vi "Phased array GUI.vi"() -> ()   [LabVIEW 2020]
uses:
  <vilib>/Instr/_visa.llb/Select Event Type.ctl
  Devices/Controls/Register to Write.ctl
  <vilib>/Instr/_visa.llb/VISA Configure Serial Port (Instr).vi
  <vilib>/Utility/file.llb/Read Delimited Spreadsheet (string).vi
  Devices/PIC-device/PIC-Device.lvclass
panel:
  out "Array 2":string[][](array[string])
  out "Array":string[](array[string])
  in  "System Open Button":bool
  in  "Calibration data (hex)":string[][](array[string])=[["0", "1", "0", "1"], ["F", "0", "D", "0"], ["C", "6", "E", "4"], ["3", "0", "2", "0"], ["8", "3", "B", "0"], ["C", "6", "8", "8"], ["4", "0", "1", "0"], ["8", "3", "8", "3"], ["D", "7", "C", "8"], ["4", "0", "1", "1"], ["8", "3", "D", "0"], ["B", "7", "9", "A"]]
  in  "COM-port U5 & U7":refnum<visa-resource-name>
  in  "COM-port U1 & U3":refnum<visa-resource-name>
  in  "System Stop Button":bool
  in  "U3 setting":i32(slide) min=0 max=180 step=90 scale=0.0..180.0
  in  "U7 setting":i32(slide) min=0 max=180 step=90 scale=0.0..180.0
  in  "U5 setting":i32(slide) min=0 max=180 step=90 scale=0.0..180.0
  in  "U1 setting":i32(slide) min=0 max=180 step=90 scale=0.0..180.0
  in  "Setting":i32[][](array[numeric])=[[1, 0, 0, 0, 0, 0], [1, 90, 0, 0, 0, 0], [1, 180, 0, 0, 0, 0], [3, 0, 0, 0, 0, 0], [3, 90, 0, 0, 0, 0], [3, 180, 0, 0, 0, 0], [5, 0, 0, 0, 0, 0], [5, 90, 0, 0, 0, 0], [5, 180, 0, 0, 0, 0], [7, 0, 0, 0, 0, 0], [7, 90, 0, 0, 0, 0], [7, 180, 0, 0, 0, 0]]
  # "Ux     angle    C1     C2     C3     C4"
  # "U1"
  # "U5"
  # "U3"
  # "U7"
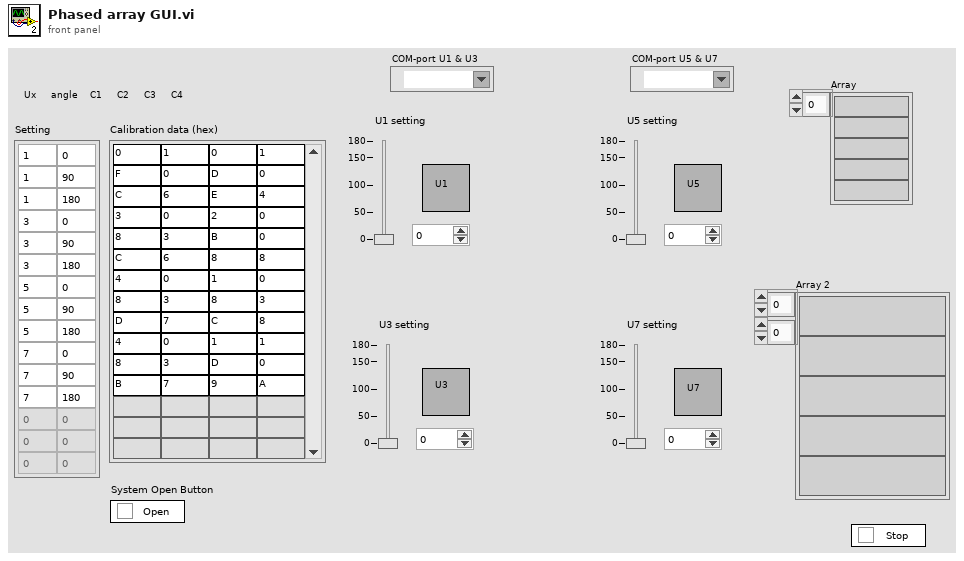
[diagram p1: front panel]
types:
  T1 = typedef "Select Event Type.ctl" = u32
  T2 = typedef "PIC-Device.lvclass/Register to Write.ctl" = cluster{"Register":u32, "Value":u32, "Dev Address":u32, "Physical Adress":u32}
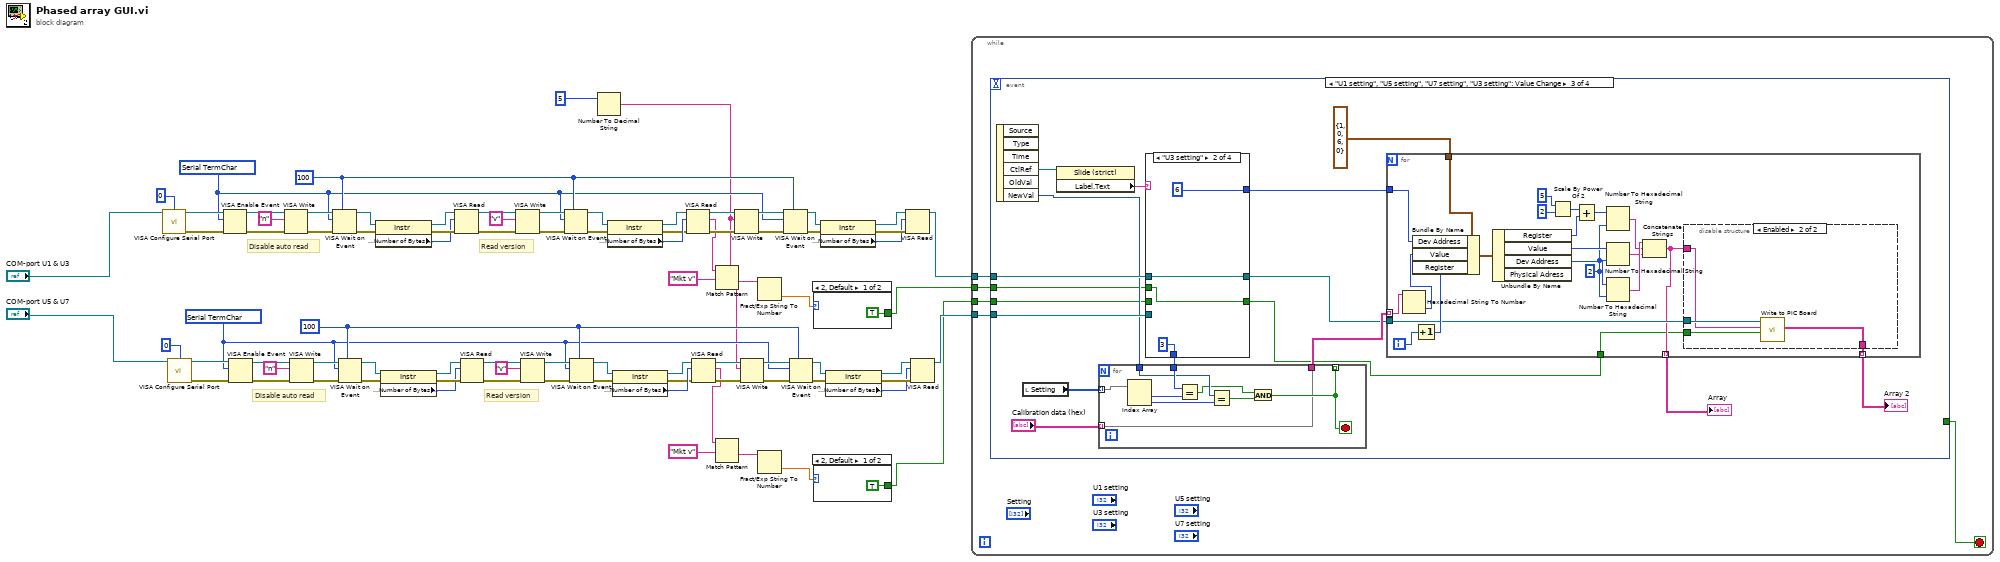
[diagram p0: block diagram]
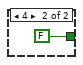
[diagram p2: hidden frame]
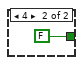
[diagram p3: hidden frame]
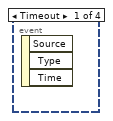
[diagram p4: hidden frame]
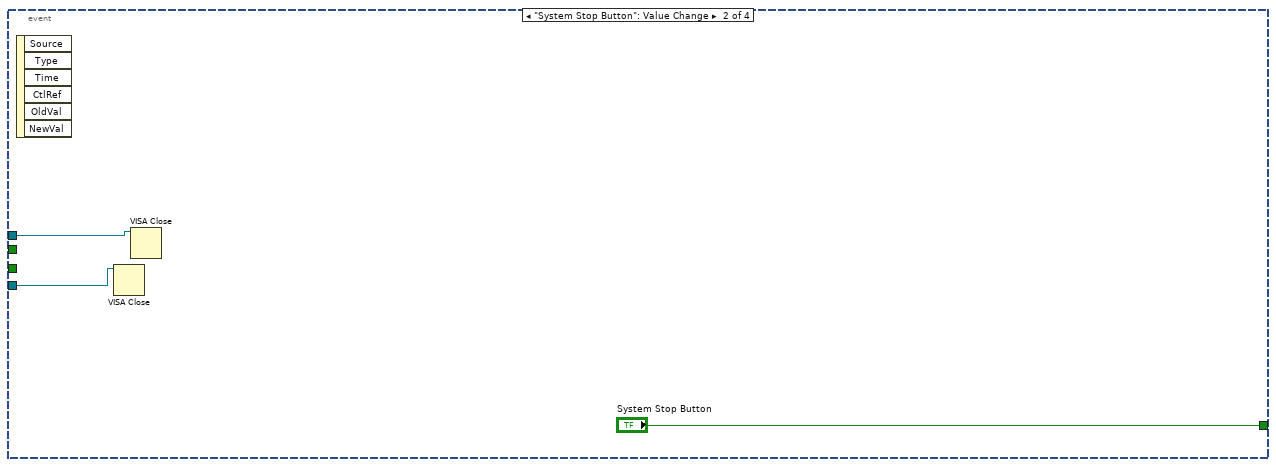
[diagram p5: hidden frame]
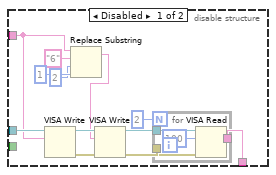
[diagram p6: hidden frame]
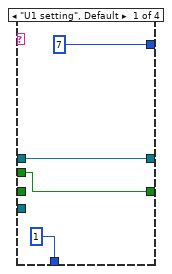
[diagram p7: hidden frame]
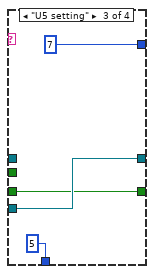
[diagram p8: hidden frame]
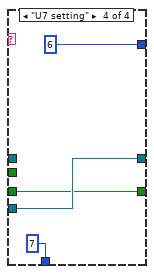
[diagram p9: hidden frame]
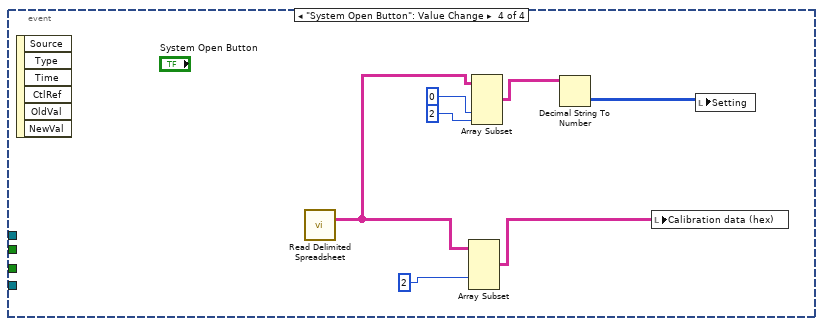
[diagram p10: hidden frame]
diagram:
  w18 = u32 100 ("timeout (0)")
  w17 = T1 1073684516 items=["Service Request"=1073684491, "Trigger"=3221168138, "Clear"=1073684493, "VXI Signal"=1073684512, "VXI/VME Interrupt"=3221168161, "VXI/VME Sysfail"=1073684509, "VXI/VME Sysreset"=1073684510, "GPIB CIC"=1073684498, "GPIB Talk"=1073684499, "GPIB Listen"=1073684500, "PXI Interrupt"=1073684514, "Serial Break"=1073684515, "Serial TermChar"=1073684516, "Serial CTS"=1073684521, "Serial DSR"=1073684522, "Serial DCD"=1073684524, "Serial RI"=1073684526, "Serial Character"=1073684533, "USB Interrupt"=1073684535, "All Enabled"=1073709055] ("Event Type")
  w52 = u32 100 ("timeout (0)")
  w51 = T1 1073684516 items=["Service Request"=1073684491, "Trigger"=3221168138, "Clear"=1073684493, "VXI Signal"=1073684512, "VXI/VME Interrupt"=3221168161, "VXI/VME Sysfail"=1073684509, "VXI/VME Sysreset"=1073684510, "GPIB CIC"=1073684498, "GPIB Talk"=1073684499, "GPIB Listen"=1073684500, "PXI Interrupt"=1073684514, "Serial Break"=1073684515, "Serial TermChar"=1073684516, "Serial CTS"=1073684521, "Serial DSR"=1073684522, "Serial DCD"=1073684524, "Serial RI"=1073684526, "Serial Character"=1073684533, "USB Interrupt"=1073684535, "All Enabled"=1073709055] ("Event Type")
  # "Read version"
  # "Disable auto read"
  # "Read version"
  # "Disable auto read"
  n1 = call-poly "VISA Configure Serial Port"("VISA resource name"="COM-port U1 & U3", "termination char\n(0xA = '\\n' = LF)"=u8 0 ("termination char\n(0xA = '\\n' = LF)")) -> ("VISA resource name out"=w48:refnum<visa-resource-name>, "error out"=w49:errorcluster)  [unwired: 12 in]
  n2 = call-poly "VISA Configure Serial Port"("VISA resource name"="COM-port U5 & U7", "termination char\n(0xA = '\\n' = LF)"=u8 0 ("termination char\n(0xA = '\\n' = LF)")) -> ("VISA resource name out"=w82:refnum<visa-resource-name>, "error out"=w83:errorcluster)  [unwired: 12 in]
  n3 = VISA Enable Event(8:w49, 10:w17, 11:w48) -> (0:w47:errorcluster, 3:w46:refnum<visa-resource-name>)  [unwired: 1 in]
  n4 = VISA Enable Event(8:w83, 10:w51, 11:w82) -> (0:w81:errorcluster, 3:w80:refnum<visa-resource-name>)  [unwired: 1 in]
  n5 = VISA Write(VISA resource name=w46, write buffer="n", error in (no error)=w47) -> (VISA resource name out=w43:refnum<visa-resource-name>, error out=w44:errorcluster)  [unwired: 1 out]
  n6 = VISA Write(VISA resource name=w80, write buffer="n", error in (no error)=w81) -> (VISA resource name out=w77:refnum<visa-resource-name>, error out=w78:errorcluster)  [unwired: 1 out]
  n7 = VISA Wait on Event(7:w18, 8:w44, 10:w17, 11:w43) -> (0:w41:errorcluster, 3:w42:refnum<visa-resource-name>)  [unwired: 1 in, 2 out]
  n8 = VISA Wait on Event(7:w52, 8:w78, 10:w51, 11:w77) -> (0:w75:errorcluster, 3:w76:refnum<visa-resource-name>)  [unwired: 1 in, 2 out]
  n9 = property class="Instr"(reference=w42, error in=w41) -> (reference out=w38:refnum<visa-resource-name>, error out=w40:errorcluster, "Serial Settings:Number of Bytes at Serial Port"=w39:u32)
  n10 = property class="Instr"(reference=w76, error in=w75) -> (reference out=w72:refnum<visa-resource-name>, error out=w74:errorcluster, "Serial Settings:Number of Bytes at Serial Port"=w73:u32)
  n11 = VISA Read(VISA resource name=w38, byte count=w39, error in (no error)=w40) -> (VISA resource name out=w22:refnum<visa-resource-name>, error out=w21:errorcluster)  [unwired: 2 out]
  n12 = VISA Read(VISA resource name=w72, byte count=w73, error in (no error)=w74) -> (VISA resource name out=w56:refnum<visa-resource-name>, error out=w55:errorcluster)  [unwired: 2 out]
  n13 = VISA Write(VISA resource name=w22, write buffer="v", error in (no error)=w21) -> (VISA resource name out=w25:refnum<visa-resource-name>, error out=w24:errorcluster)  [unwired: 1 out]
  n14 = VISA Write(VISA resource name=w56, write buffer="v", error in (no error)=w55) -> (VISA resource name out=w59:refnum<visa-resource-name>, error out=w58:errorcluster)  [unwired: 1 out]
  n15 = VISA Wait on Event(7:w18, 8:w24, 10:w17, 11:w25) -> (0:w27:errorcluster, 3:w26:refnum<visa-resource-name>)  [unwired: 1 in, 2 out]
  n16 = VISA Wait on Event(7:w52, 8:w58, 10:w51, 11:w59) -> (0:w61:errorcluster, 3:w60:refnum<visa-resource-name>)  [unwired: 1 in, 2 out]
  n17 = Number To Decimal String(number=5) -> (decimal integer string=w11:string)  [unwired: 1 in]
  n18 = property class="Instr"(reference=w26, error in=w27) -> (reference out=w30:refnum<visa-resource-name>, error out=w28:errorcluster, "Serial Settings:Number of Bytes at Serial Port"=w29:u32)
  n19 = property class="Instr"(reference=w60, error in=w61) -> (reference out=w64:refnum<visa-resource-name>, error out=w62:errorcluster, "Serial Settings:Number of Bytes at Serial Port"=w63:u32)
  n20 = VISA Read(VISA resource name=w30, byte count=w29, error in (no error)=w28) -> (VISA resource name out=w19:refnum<visa-resource-name>, read buffer=w3:string, error out=w20:errorcluster)  [unwired: 1 out]
  n21 = VISA Read(VISA resource name=w64, byte count=w63, error in (no error)=w62) -> (VISA resource name out=w53:refnum<visa-resource-name>, read buffer=w7:string, error out=w54:errorcluster)  [unwired: 1 out]
  n22 = Match Pattern(string=w3, regular expression="Mkt v" ("format string")) -> (after substring=w5:string)  [unwired: 1 in, 3 out]
  n23 = Match Pattern(string=w7, regular expression="Mkt v" ("format string")) -> (after substring=w9:string)  [unwired: 1 in, 3 out]
  n24 = VISA Write(VISA resource name=w19, write buffer=w11, error in (no error)=w20) -> (VISA resource name out=w36:refnum<visa-resource-name>, error out=w37:errorcluster)  [unwired: 1 out]
  n25 = VISA Write(VISA resource name=w53, write buffer=w11, error in (no error)=w54) -> (VISA resource name out=w70:refnum<visa-resource-name>, error out=w71:errorcluster)  [unwired: 1 out]
  n26 = Fract/Exp String To Number(string=w5) -> (number=w6:dbl)  [unwired: 3 in, 1 out]
  n27 = Fract/Exp String To Number(string=w9) -> (number=w8:dbl)  [unwired: 3 in, 1 out]
  n28 = VISA Wait on Event(7:w18, 8:w37, 10:w17, 11:w36) -> (0:w34:errorcluster, 3:w35:refnum<visa-resource-name>)  [unwired: 1 in, 2 out]
  n29 = VISA Wait on Event(7:w52, 8:w71, 10:w51, 11:w70) -> (0:w68:errorcluster, 3:w69:refnum<visa-resource-name>)  [unwired: 1 in, 2 out]
  n30 = case shown="2, Default" w6 {
    tunnel: [TRUE FALSE] -> w2
    frame 2, Default {
    }
    frame 4 {
    }
  }
  n31 = case shown="2, Default" w8 {
    tunnel: [TRUE FALSE] -> w1
    frame 2, Default {
    }
    frame 4 {
    }
  }
  n32 = property class="Instr"(reference=w35, error in=w34) -> (reference out=w31:refnum<visa-resource-name>, error out=w33:errorcluster, "Serial Settings:Number of Bytes at Serial Port"=w32:u32)
  n33 = property class="Instr"(reference=w69, error in=w68) -> (reference out=w65:refnum<visa-resource-name>, error out=w67:errorcluster, "Serial Settings:Number of Bytes at Serial Port"=w66:u32)
  n34 = VISA Read(VISA resource name=w31, byte count=w32, error in (no error)=w33) -> (VISA resource name out=w13:refnum<visa-resource-name>)  [unwired: 3 out]
  n35 = VISA Read(VISA resource name=w65, byte count=w66, error in (no error)=w67) -> (VISA resource name out=w14:refnum<visa-resource-name>)  [unwired: 3 out]
  n36 = while {
    tunnel: w13 -> [w92]
    tunnel: w14 -> [w91]
    tunnel: w2 -> [w90]
    tunnel: w1 -> [w89]
    stop <- w93 stop-if-true
    n37 = event shown="[2] \"U1 setting\", \"U5 setting\", \"U7 setting\", \"U3 setting\": Value Change" {
      selector: _ -> [_ _ _ _]
      dyn-events: _ -> [_ _ _ _]
      timeout: _ -> [_ _ _ _]
      tunnel: [_ "System Stop Button" _ _] -> w93
      tunnel: w92 -> [_ w95 w111 _]
      tunnel: w91 -> [_ w94 w110 _]
      tunnel: w90 -> [_ _ w99 _]
      tunnel: w89 -> [_ _ w98 _]
      event Timeout {
        n38 = event-data() -> ()  [unwired: 1 in, 3 out]
      }
      event "System Stop Button": Value Change {
        n39 = event-data() -> ()  [unwired: 1 in, 6 out]
        n40 = VISA Close(VISA resource name=w94) -> ()  [unwired: 1 in, 1 out]
        n41 = VISA Close(VISA resource name=w95) -> ()  [unwired: 1 in, 1 out]
      }
      event "U1 setting", "U5 setting", "U7 setting", "U3 setting": Value Change {
        n42 = event-data() -> ("CtlRef"=w113:refnum<vi>, "NewVal"=w107:i32)  [unwired: 1 in, 4 out]
        n43 = local read "Setting"() -> (w109:i32[][])
        n44 = property class="Slide (strict)"(reference=w113) -> ("Label.Text"=w112:string)  [unwired: 1 in, 2 out]
        n45 = case shown="\"U3 setting\"" w112 {
          tunnel: [w168 w172 w175 w179] -> w102
          tunnel: w111 -> [w168 w172 _ _]
          tunnel: [u32 7 ("Dev Address") u32 6 ("Dev Address") u32 7 ("Dev Address") u32 6 ("Dev Address")] -> w103
          tunnel: w110 -> [_ _ w175 w179]
          tunnel: [1 3 5 7] -> w108
          tunnel: w99 -> [w165 w169 _ _]
          tunnel: w98 -> [_ _ w173 w177]
          tunnel: [w165 w169 w173 w177] -> w97
          frame "U1 setting", Default {
          }
          frame "U3 setting" {
          }
          frame "U5 setting" {
          }
          frame "U7 setting" {
          }
        }
        n46 = for {
          tunnel: w109 -> [w164] mode=indexing
          tunnel: w108 -> [w162]
          tunnel: w107 -> [w160]
          tunnel: [w157] -> _ mode=indexing
          tunnel: [w156] -> w105
          tunnel: "Calibration data (hex)" -> [w156] mode=indexing
          stop <- w157 stop-if-true
          n47 = Index Array(array=w164) -> (element #1=w163:i32, element #2=w161:i32)  [unwired: 2 in]
          n48 = Equal?(x=w162, y=w163) -> (x = y?=w158:bool)
          n49 = Equal?(x=w160, y=w161) -> (x = y?=w159:bool)
          n50 = And(x=w158, y=w159) -> (x .and. y?=w157:bool)
        }
        n51 = for {
          tunnel: w105 -> [w131] mode=indexing
          tunnel: T2 {"Register"=1, "Value"=0, "Dev Address"=6, "Physical Adress"=0} ("Register to Write") -> [w134]
          tunnel: w103 -> [w132]
          tunnel: w102 -> [w117]
          tunnel: [w115] -> w101 mode=indexing
          tunnel: [w116] -> w100 mode=indexing
          tunnel: w97 -> [w114]
          i -> [w135]
          w122 = i16 2 ("width (-)")
          n52 = Hexadecimal String To Number(string=w131) -> (number=w130:u32)  [unwired: 2 in, 1 out]
          n53 = Increment(x=w135) -> (x+1=w133:i32)
          n54 = Bundle By Name(cluster=w134, "Dev Address"=w132, "Value"=w130, "Register"=w133) -> (w118:T2)
          n55 = Unbundle By Name(w118) -> ("Register"=w126:u32, "Value"=w124:u32, "Dev Address"=w123:u32)  [unwired: 1 out]
          n56 = Scale By Power Of 2(n=u32 5, x=u32 2) -> (x*2^n=w127:u32)
          n57 = Add(x=w127, y=w126) -> (x+y=w125:u32)
          n58 = Number To Hexadecimal String(1:w122, 2:w125) -> (0:w120:string)
          n59 = Number To Hexadecimal String(1:w122, 2:w124) -> (0:w119:string)
          n60 = Number To Hexadecimal String(1:w122, 2:w123) -> (0:w121:string)
          n61 = Concatenate Strings(w121, w120, w119) -> (w115:string)
          n62 = disable-structure shown="Enabled" {
            disable-tunnel: w115 -> [w136 w154]
            disable-tunnel: w117 -> [w147 w155]
            disable-tunnel: [w144 w153] -> w116
            disable-tunnel: w114 -> [_ w152]
            frame Disabled {
              n63 = VISA Write(VISA resource name=w147, write buffer=w136) -> (VISA resource name out=w143:refnum<visa-resource-name>, error out=w145:errorcluster)  [unwired: 1 in, 1 out]
              n64 = Replace Substring(2:1 ("length (len. of substring)"), 3:2 ("offset (0)"), 4:"6" ("substring (\"\")"), 5:w136) -> (1:w137:string)  [unwired: 1 out]
              n65 = VISA Write(VISA resource name=w143, write buffer=w137, error in (no error)=w145) -> (VISA resource name out=w142:refnum<visa-resource-name>, error out=w146:errorcluster)  [unwired: 1 out]
              n66 = for {
                N: 2 -> [_]
                tunnel: w146 -> [w151]
                tunnel: [w150] -> w144
                tunnel: w142 -> [w149]
                n67 = VISA Read(VISA resource name=w149, byte count=u32 100, error in (no error)=w151) -> (read buffer=w150:string)  [unwired: 3 out]
              }
            }
            frame Enabled {
              n68 = call "Write to PIC Board.vi"("Ignore address in return"=w152, "String to write"=w154, "VISA Refnum in"=w155) -> ("Return"=w153:string[])  [unwired: 7 in, 1 out]
            }
          }
        }
        "Array" <- w101
        "Array 2" <- w100
      }
      event "System Open Button": Value Change {
        n69 = event-data() -> ()  [unwired: 1 in, 6 out]
        n70 = call-poly <vilib>:"Read Delimited Spreadsheet.vi"() -> ("all rows"=w186:string[][])  [unwired: 10 in, 5 out]
        n71 = Array Subset(array=w186, index (col)=2 ("index")) -> (w187:string[][])  [unwired: 3 in]
        n72 = Array Subset(array=w186, index (col)=0 ("index"), length (col)=2 ("length")) -> (w185:string[][])  [unwired: 2 in]
        n73 = Decimal String To Number(string=w185) -> (number=w184:i32[][])  [unwired: 2 in, 1 out]
        n74 = local write "Calibration data (hex)"(w187) -> ()
        n75 = local write "Setting"(w184) -> ()
      }
    }
  }
